vi "Constants.vi"() -> ()   [LabVIEW 2013]
panel:
  in  "NoChange.Syntax":string="Unchanged"
  in  "Menu.StepPrefix":string="Step."
  in  "Ramp.Syntax":string="Ramp (Value, Duration)"
  in  "Step.Syntax":string="Step (Value)"
  in  "# of Static Columns":u32=3
  in  "Menu.ChannelPrefix":string="Channel."
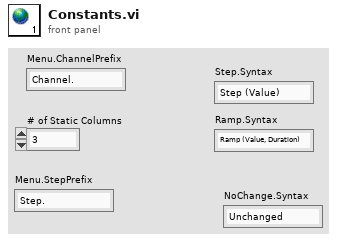
[diagram p1: front panel]
diagram:
